vi "Conversor de sinais.vi"(3 "Sinal a2":string, 4 "Sinal a1":string, 5 "Sinal a0":string) -> (0 "Sinal a2":i32, 1 "Sinal a1":i32, 2 "Sinal a0":i32)   [LabVIEW 2014]
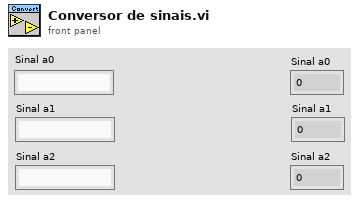
[diagram p1: front panel]
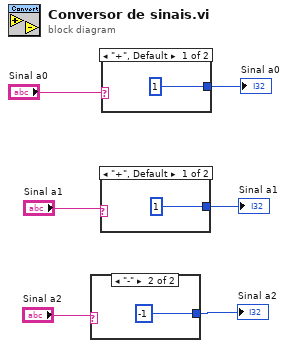
[diagram p0: block diagram]
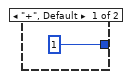
[diagram p2: hidden frame]
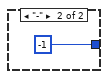
[diagram p3: hidden frame]
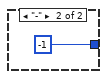
[diagram p4: hidden frame]
diagram:
  n1 = case shown="\"-\"" "Sinal a2" {
    tunnel: [1 -1] -> w1
    frame "+", Default {
    }
    frame "-" {
    }
  }
  "Sinal a2" <- w1
  n2 = case shown="\"+\", Default" "Sinal a1" {
    tunnel: [1 -1] -> w4
    frame "+", Default {
    }
    frame "-" {
    }
  }
  "Sinal a1" <- w4
  n3 = case shown="\"+\", Default" "Sinal a0" {
    tunnel: [1 -1] -> w3
    frame "+", Default {
    }
    frame "-" {
    }
  }
  "Sinal a0" <- w3
